vi "Start Stop.vi"(6 "ms Delay (-1=No change)":i32=-1, 8 "error in (no error)":errorcluster, 9 "Start? (T)":bool=TRUE, 10 "Timer Message":string, 11 "Queue in":refnum<queue>) -> (0 "error out":errorcluster, 3 "Queue out":refnum<queue>)   [LabVIEW 2021, in "QueueTimer.lvlib"]
doc: "Start or stop a specific queue timer specified by the <b>Timer Message</b>. Optionally, specify the <b>ms Delay</b> to update the periodic delay to enqueue (-1=No change).\n\nNote: Queue timers are uniquely identified by the `<queue>+<timer_message>`."
uses:
  QueueTimer.lvlib
  <vilib>/Utility/error.llb/Error Cluster From Error Code.vi
  <vilib>/ErrorRing/Error Ring.xnode
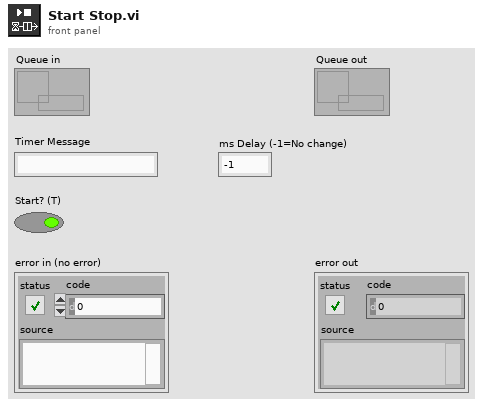
[diagram p1: front panel]
types:
  T1 = cluster{"Emit":refnum<queue>, "Time":refnum<data-value>, "Daemon":refnum<vi>}
  T2 = typedef "Queue.lvlib/Timer.ctl" = cluster{"Delay":i32, "Start":bool, "Ticks":u32}
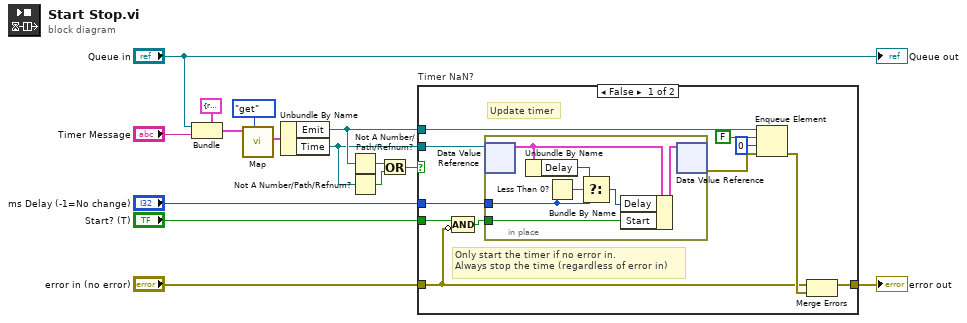
[diagram p0: block diagram]
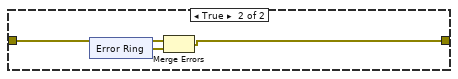
[diagram p2: hidden frame]
diagram:
  n1 = Bundle(cluster=cluster{"Queue":refnum<queue>, "Message":string} {"Queue"=refnum, "Message"=""} ("Timer Id"), "Queue"="Queue in", "Message"="Timer Message") -> (w2:cluster{"Queue":refnum<queue>, "Message":string})
  n2 = call "Map.vi"("Action"=enum8{"noop", "get", "set", "pop"}."get", "Timer Id"=w2) -> ("Timer out"=w6:T1)  [unwired: 7 in, 2 out]
  n3 = Unbundle By Name(w6) -> ("Emit"=w4:refnum<queue>, "Time"=w3:refnum<data-value>)
  n4 = Not A Number/Path/Refnum?(number/path/refnum=w4) -> (NaN/Path/Refnum?=w8:bool)
  n5 = Not A Number/Path/Refnum?(number/path/refnum=w3) -> (NaN/Path/Refnum?=w7:bool)
  n6 = Or(x=w8, y=w7) -> (x .or. y?=w1:bool)
  n7 = case "Timer NaN?" shown="False" w1 {
    tunnel: w4 -> [w19 _]
    tunnel: w3 -> [w26 _]
    tunnel: "error in (no error)" -> [w16 w36]
    tunnel: [w22 w35] -> w14
    tunnel: "ms Delay (-1=No change)" -> [w21 _]
    tunnel: "Start? (T)" -> [w20 _]
    frame False {
      # "Only start the timer if no error in.\nAlways stop the time (regardless of error in)"
      # "Update timer"
      n8 = Compound Arithmetic op=AND(w20, invert w16) -> (w17:bool)
      n9 = in-place {
        in-place-border: w21 -> [w27]
        in-place-border: w17 -> [w32]
        n10 = in-place-dvr #1(w26) -> (w31:T2)  [unwired: 1 out]
        n11 = Unbundle By Name(w31) -> ("Delay"=w29:i32)
        n12 = Less Than 0?(x=w27) -> (x < 0?=w30:bool)
        n13 = Select(t=w29, s=w30, f=w27) -> (s? t:f=w28:i32)
        n14 = Bundle By Name(cluster=w31, "Delay"=w28, "Start"=w32) -> (w33:T2)
        n15 = in-place-dvr #1(w33) -> (w24:errorcluster)  [unwired: 1 out]
      }
      n16 = Enqueue Element(queue=w19, element=FALSE, timeout in ms (-1)=0, error in (no error)=w24) -> (error out=w23:errorcluster)  [unwired: 2 out]
      n17 = Merge Errors(w16, w23) -> (w22:errorcluster)
    }
    frame True {
      n18 = xnode "Error Ring"() -> ("error out"=w34:errorcluster)
      n19 = Merge Errors(w36, w34) -> (w35:errorcluster)
    }
  }
  "error out" <- w14
  "Queue out" <- "Queue in"
